vi "REPORT - Autofrettage.vi"(8 "error in (no error)":errorcluster, 11 "TDMS file path":path) -> ()   [LabVIEW 2025]
uses:
  <vilib>/printing/EasyPrintingControls.llb/contents.ctl
  <vilib>/Utility/NIReport.llb/Report Type (with Quick Print).ctl
  <vilib>/printing/EasyPrinting.llb/Print VI Panel or Documentation (path).vi
  <vilib>/Utility/NIReport.llb/NI_report.lvclass
  <vilib>/Utility/NIReport.llb/NI_ReportGenerationCore.lvlib
panel:
  out "graph":cluster{"X":dbl[], "Y":dbl[]}[](graph)
  out "Operator:":string
  out "String":string
  in  "Notes":string
  out "Test Date:":dbl format="%<%x>T"
  out "Test ID:":string
  out "Part Number:":string
  out "Job Number:":string
  # "Autofrettage Report"
  # "Unit Under Test"
  # "Test Result"
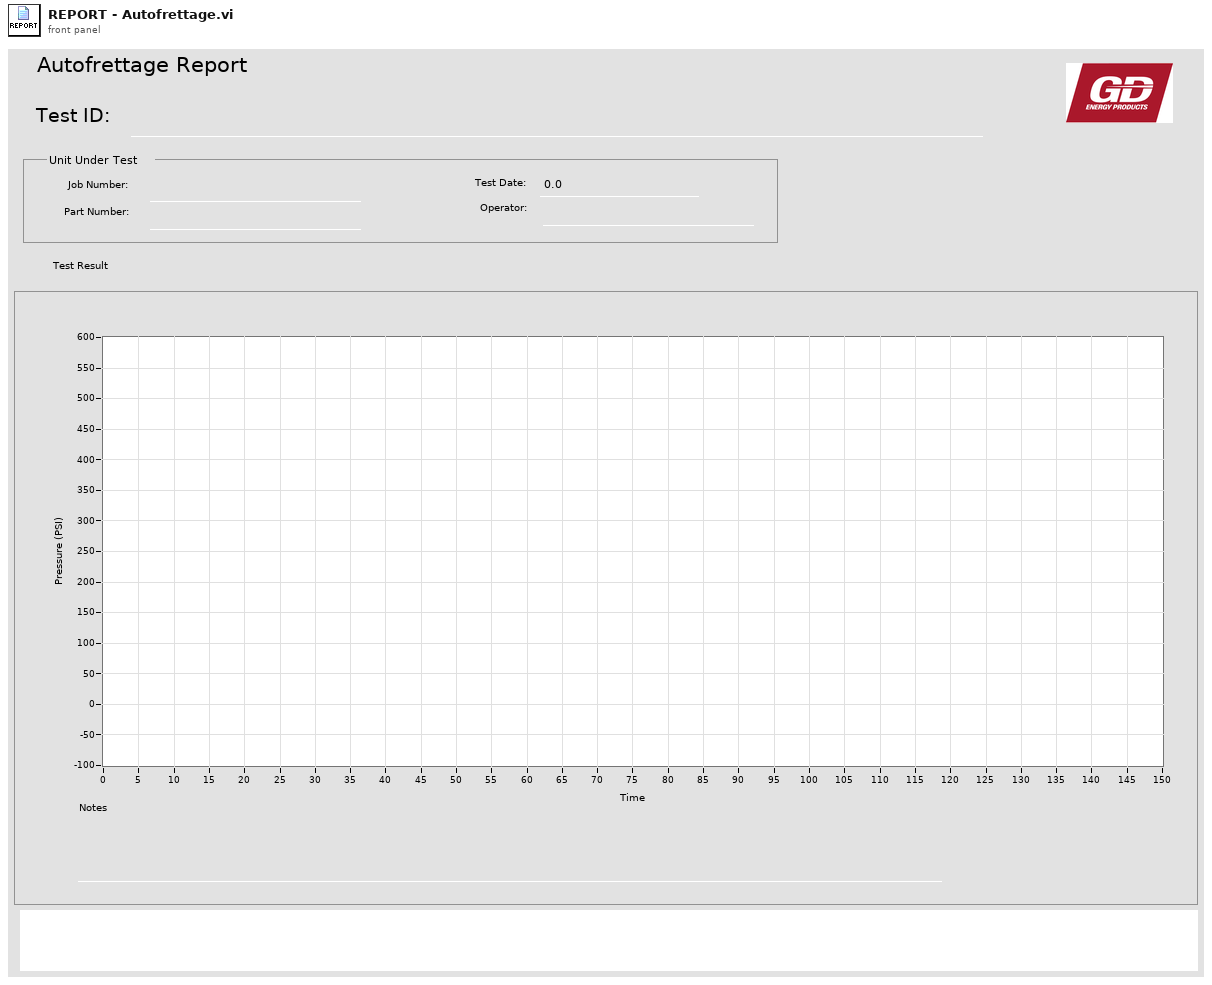
[diagram p1: front panel]
types:
  T1 = typedef "NI_ReportGenerationCore.lvlib/Report Type (with Quick Print).ctl" = enum16{"Quick Print", "HTML", "Word", "Excel"}
  T2 = typedef "NI_ReportGenerationCore.lvlib/contents.ctl" = u16
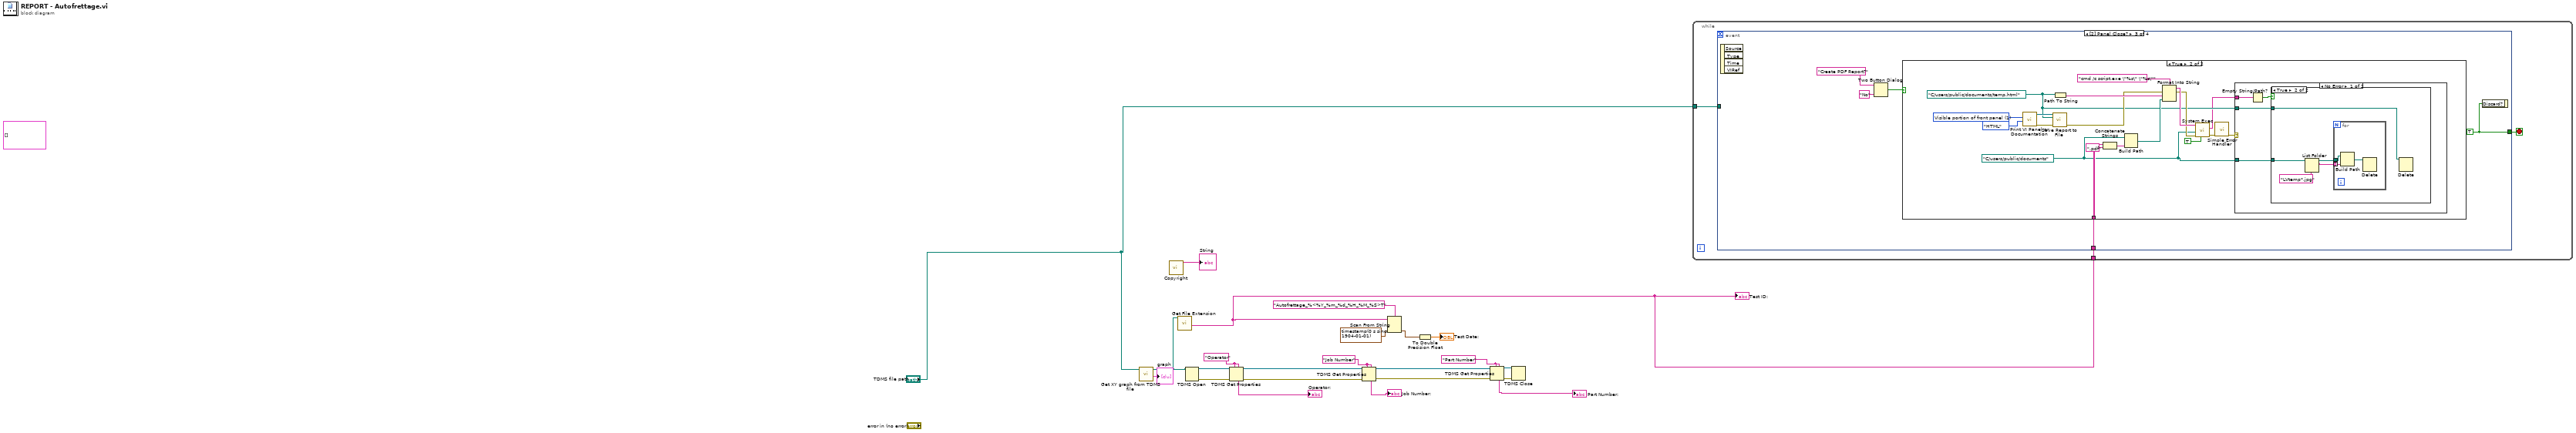
[diagram p0: block diagram]
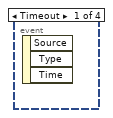
[diagram p2: hidden frame]
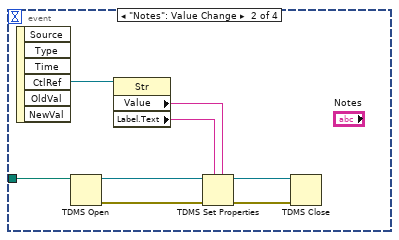
[diagram p3: hidden frame]
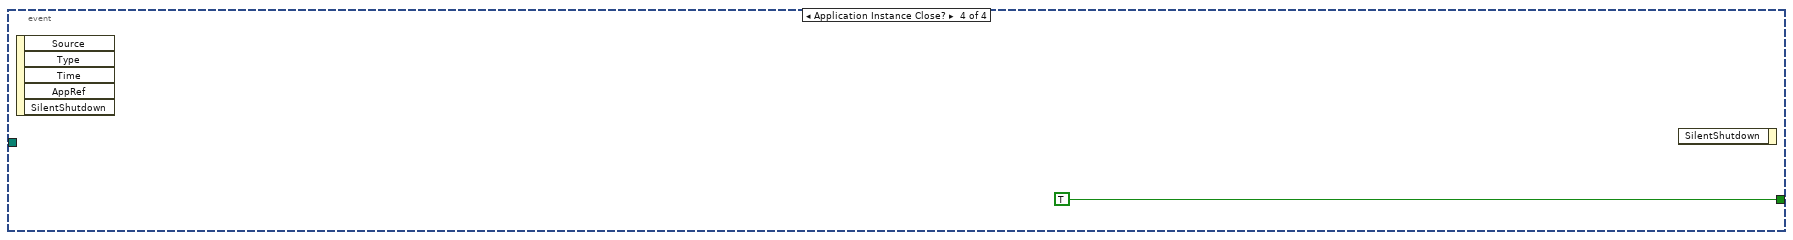
[diagram p7: hidden frame]
diagram:
  w9 = "Part Number" ("channel name")
  w11 = "Job Number" ("channel name")
  w7 = "Operator" ("channel name")
  (unwired) cluster{"X":dbl[], "Y":dbl[]}[] [] ("Restoring Force")
  n1 = call "Get XY graph from TDMS file.vi"("TDMS file path"="TDMS file path") -> ("graph"=→"graph":cluster{"X":dbl[], "Y":dbl[]}[], "TDMS file path out"=w4:path)  [unwired: 8 in, 1 out]
  n2 = call "Copyright.vi"() -> ("String"=→"String":string)  [unwired: 11 in]
  n3 = call <vilib>:"Get File Extension.vi"("file"=w4) -> ("filename without extension"=w1:string)  [unwired: 6 in, 4 out]
  "Test ID:" <- w1
  n4 = TDMS Open(11:w4) -> (0:w16:errorcluster, 3:w21:refnum<k34>)  [unwired: 6 in]
  n5 = TDMS Get Properties(5:w7, 7:w7, 8:w16, 11:w21) -> (0:w17:errorcluster, 3:w20:refnum<k34>, 4:→"Operator:":string)  [unwired: 2 in, 3 out]
  n6 = TDMS Get Properties(5:w11, 7:w11, 8:w17, 11:w20) -> (0:w18:errorcluster, 3:w19:refnum<k34>, 4:→"Job Number:":string)  [unwired: 2 in, 3 out]
  n7 = Scan From String(format string="Autofrettage_%<%Y_%m_%d_%H_%M_%S>T", input string=w1, default 1=timestamp(0 s since 1904-01-01)) -> (output 1=w13:timestamp)  [unwired: 2 in, 3 out]
  n8 = To Double Precision Float(number=w13) -> (double precision float=→"Test Date:":dbl)
  n9 = TDMS Get Properties(5:w9, 7:w9, 8:w18, 11:w19) -> (0:w3:errorcluster, 3:w2:refnum<k34>, 4:→"Part Number:":string)  [unwired: 2 in, 3 out]
  n10 = TDMS Close(8:w3, 11:w2) -> ()  [unwired: 2 out]
  n11 = while {
    tunnel: "TDMS file path" -> [w25]
    tunnel: w1 -> [w24]
    stop <- w26 stop-if-true
    n12 = event shown="[2] Panel Close?" {
      selector: _ -> [_ _ _ _]
      dyn-events: _ -> [_ _ _ _]
      timeout: _ -> [_ _ _ _]
      tunnel: [_ _ w39 TRUE] -> w26
      tunnel: w25 -> [_ w34 _ _]
      tunnel: w24 -> [_ _ w35 _]
      event Timeout {
        n13 = event-data() -> ()  [unwired: 1 in, 3 out]
      }
      event "Notes": Value Change {
        n14 = event-data() -> ("CtlRef"=w32:refnum<vi>)  [unwired: 1 in, 5 out]
        n15 = TDMS Open(11:w34) -> (0:w27:errorcluster, 3:w33:refnum<k34>)  [unwired: 6 in]
        n16 = property class="Str"(reference=w32) -> ("Value"=w29:string, "Label.Text"=w30:string)  [unwired: 1 in, 2 out]
        n17 = TDMS Set Properties(5:w29, 7:w30, 8:w27, 11:w33) -> (0:w28:errorcluster, 3:w31:refnum<k34>)  [unwired: 2 in, 2 out]
        n18 = TDMS Close(8:w28, 11:w31) -> ()  [unwired: 2 out]
      }
      event Panel Close? {
        w39 = TRUE
        n19 = event-data() -> ()  [unwired: 1 in, 4 out]
        n20 = Two Button Dialog(message="Create PDF Report?", 1:"No" ("F button name (\"Cancel\")")) -> (T button?=w36:bool)  [unwired: 1 in]
        n21 = case shown="True" w36 {
          tunnel: w35 -> [_ w47]
          frame False {
          }
          frame True {
            w43 = path "C:/users/public/documents" ("working directory")
            w53 = T2 1 items=["Complete front panel", "Visible portion of front panel", "Icon, description, panel and diagram", "Documentation: Using the panel", "Documentation: Using as a subVI", "Documentation: Complete", "Documentation: Custom"] ("contents (complete front panel)")
            w42 = path "C:/users/public/documents/temp.html" ("report file path")
            n22 = call-poly <vilib>:"Print VI Panel or Documentation.vi"("report type (Quick Print)"=Report_Type_(with_Quick_Print)."HTML", "contents (complete front panel)"=w53) -> ("error out"=w50:errorcluster, "report out"=w56:refnum<class "NI_report.lvclass">)  [unwired: 8 in]
            n23 = call-dynamic "Save Report to File.vi"("report in"=w56, "report file path"=w42, "error in (no error)"=w50) -> ("error out"=w44:errorcluster)  [unwired: 11 in, 1 out]
            n24 = Path To String(path=w42) -> (string=w57:string)
            n25 = Concatenate Strings(w47, ".pdf" ("string")) -> (w48:string)
            n26 = Build Path(base path=w43, name or relative path=w48) -> (appended path=w45:path)
            n27 = Format Into String(format string="cmd /c script.exe \"%s\" \"%s\"" ("command line"), error in=w44, w57, w45) -> (resulting string=w58:string, error out=w51:errorcluster)  [unwired: 1 in]
            n28 = call <vilib>:"System Exec.vi"("run minimized? (F)"=TRUE, "error in (no error)"=w51, "working directory"=w43, "command line"=w58) -> ("error out"=w52:errorcluster, "standard error"=w40:string)  [unwired: 4 in, 2 out]
            n29 = call <vilib>:"Simple Error Handler.vi"("error in (no error)"=w52) -> ("error out"=w41:errorcluster)  [unwired: 4 in, 4 out]
            n30 = case shown="No Error" w41 {
              tunnel: w43 -> [w62 _]
              tunnel: w42 -> [w61 _]
              tunnel: w40 -> [w60 _]
              frame No Error {
                n31 = Empty String/Path?(string/path=w60) -> (empty?=w59:bool)
                n32 = case shown="True" w59 {
                  tunnel: w62 -> [_ w67]
                  tunnel: w61 -> [_ w63]
                  frame False {
                  }
                  frame True {
                    n33 = List Folder(path=w67, pattern="LVtemp*.jpg") -> (path out=w64:path, filenames=w65:string[])  [unwired: 2 in, 2 out]
                    n34 = for {
                      tunnel: w65 -> [w70] mode=indexing
                      tunnel: w64 -> [w69]
                      n35 = Build Path(base path=w69, name or relative path=w70) -> (appended path=w68:path)
                      n36 = Delete(path (use dialog)=w68) -> ()  [unwired: 4 in, 3 out]
                    }
                    n37 = Delete(path (use dialog)=w63) -> ()  [unwired: 4 in, 3 out]
                  }
                }
              }
              frame Error {
              }
            }
          }
        }
        n38 = event-data("Discard?"=w39) -> ()  [unwired: 1 in, 1 out]
      }
      event Application Instance Close? {
        n39 = event-data() -> ()  [unwired: 1 in, 5 out]
        n40 = event-data() -> ()  [unwired: 2 in, 1 out]
      }
    }
  }
